vi "Add Path.vi"(10 "Path":string, 11 "URI in":refnum<class "URI.lvclass">) -> (3 "URI out":refnum<class "URI.lvclass">)   [LabVIEW 2020, in "URI.lvlib" / "URI.lvclass"]
uses:
  URI.lvclass
  URI.lvclass/URI.ctl
  URI.lvlib
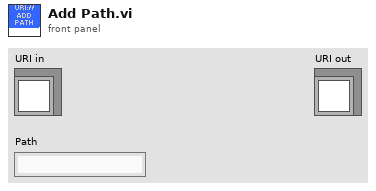
[diagram p1: front panel]
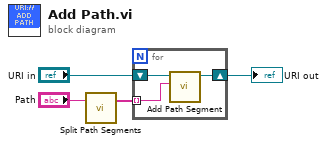
[diagram p0: block diagram]
diagram:
  n1 = call "Split Path Segments.vi"("Path String"="Path") -> ("Path Segments"=w2:string[])  [unwired: 6 in]
  n2 = for {
    shift-right: [w5] -> w1
    shift-left: "URI in" -> [w7]
    tunnel: w2 -> [w6] mode=indexing
    n3 = call "Add Path Segment.vi"("Path Segment"=w6, "URI in"=w7) -> ("URI out"=w5:refnum<class "URI.lvclass">)  [unwired: 9 in]
  }
  "URI out" <- w1
